vi "温度校准.vi"(7 "校准参数":u16(ring) caption="校准参数：" items=["pH", "DO", "浊度", "电导率", "叶绿素a", "藻密度", "ORP", "DO2", "氯化物"], 8 "error in (no error)":errorcluster caption="错误输入（无错误）", 11 "校准温度":sgl) -> (0 "error out":errorcluster caption="错误输出")   [LabVIEW 2016, in "斯坦道多参数.lvlib"]
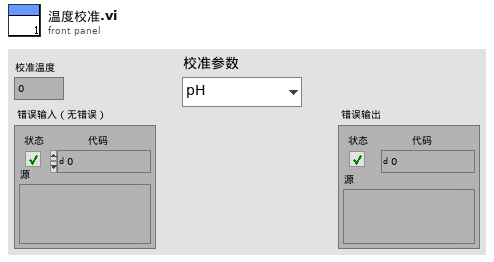
[diagram p1: front panel]
types:
  T1 = typedef "斯坦道多参数.lvlib/探头类型.ctl" = enum16{"禹山", "国弘", "纳清", "STD"}
  T2 = enum16{"null", "pH", "DO", "浊度", "电导率", "叶绿素a", "DO2", "藻密度"}
  T3 = enum16{"null", "pH", "DO", "浊度", "电导率", "叶绿素a", "DO2", "藻密度", "悬浮物"}
  T4 = enum16{"NULL", "pH", "Cond", "DO", "Turb", "ORP"}
  T5 = enum16{"NULL", "pH", "Cond", "DO", "Turb", "ORP", "6", "7", "8", "9", "氯化物"}
  T6 = enum16{"null", "pH", "DO", "浊度", "电导率", "叶绿素a", "藻密度"}
  T7 = enum16{"null", "pH", "DO", "浊度", "电导率", "叶绿素a", "藻密度", "氨氮"}
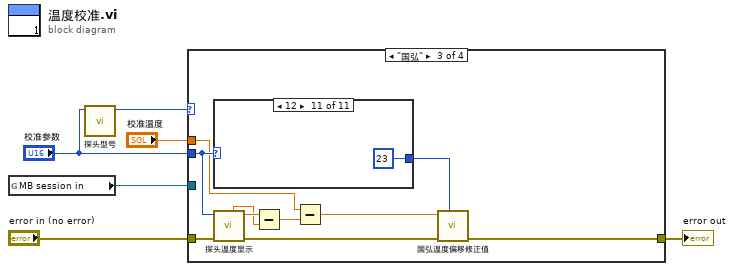
[diagram p0: block diagram]
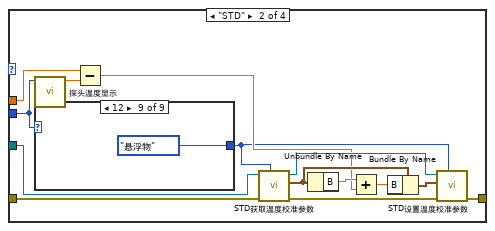
[diagram p3: hidden frame]
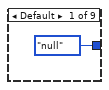
[diagram p4: hidden frame]
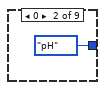
[diagram p5: hidden frame]
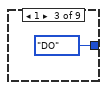
[diagram p6: hidden frame]
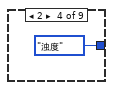
[diagram p7: hidden frame]
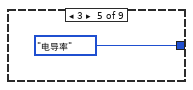
[diagram p8: hidden frame]
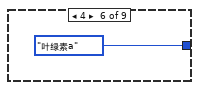
[diagram p9: hidden frame]
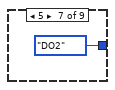
[diagram p10: hidden frame]
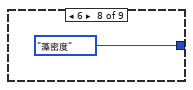
[diagram p11: hidden frame]
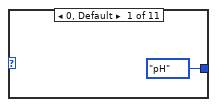
[diagram p12: hidden frame]
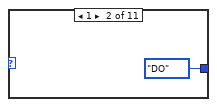
[diagram p13: hidden frame]
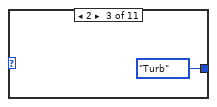
[diagram p14: hidden frame]
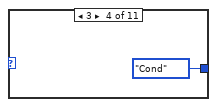
[diagram p15: hidden frame]
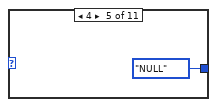
[diagram p16: hidden frame]
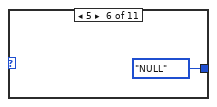
[diagram p17: hidden frame]
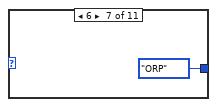
[diagram p18: hidden frame]
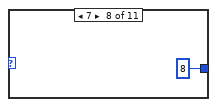
[diagram p19: hidden frame]
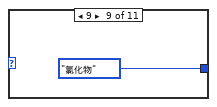
[diagram p20: hidden frame]
diagram:
  n1 = global read "多参数全局变量.vi" "MB session in"() -> (w4:refnum<class "MB_Master.lvclass">)
  n2 = call "探头型号.vi"("校准参数"="校准参数") -> ("探头型号"=w6:T1)  [unwired: 8 in, 2 out]
  n3 = case shown="\"国弘\"" w6 {
    tunnel: "校准参数" -> [_ w10 w36 w52]
    tunnel: w4 -> [_ w21 _ w54]
    tunnel: "error in (no error)" -> [w7 w8 w39 w56]
    tunnel: [w7 w11 w38 w55] -> w2
    tunnel: "校准温度" -> [_ w18 w32 w53]
    frame "禹山", Default {
    }
    frame "STD" {
      n4 = call "探头温度显示.vi"("校准参数"=w10) -> ("温度数据"=w19:sgl)  [unwired: 9 in, 1 out]
      n5 = case shown="12" w10 {
        tunnel: [T2."null" ("探头") T2."pH" ("探头") T2."DO" ("探头") T2."浊度" ("探头") T2."电导率" ("探头") T2."叶绿素a" ("探头") T2."DO2" ("探头") T2."藻密度" ("探头") T3."悬浮物" ("探头")] -> w9
        frame Default {
        }
        frame 0 {
        }
        frame 1 {
        }
        frame 2 {
        }
        frame 3 {
        }
        frame 4 {
        }
        frame 5 {
        }
        frame 6 {
        }
        frame 12 {
        }
      }
      n6 = Subtract(x=w18, y=w19) -> (x-y=w14:sgl)
      n7 = call "STD获取温度校准参数.vi"("探头"=w9, "error in (no error)"=w8, "MB session in"=w21) -> ("error out"=w17:errorcluster, "输出值"=w16:cluster{"K":sgl, "B":sgl}, "MB session out"=w20:refnum<class "MB_Master.lvclass">)  [unwired: 6 in]
      n8 = Unbundle By Name(w16) -> ("B"=w15:sgl)
      n9 = Add(x=w15, y=w14) -> (x+y=w13:sgl)
      n10 = Bundle By Name(cluster=w16, "B"=w13) -> (w12:cluster{"K":sgl, "B":sgl})
      n11 = call "STD设置温度校准参数.vi"("探头"=w9, "error in (no error)"=w17, "用户校准参数"=w12, "MB session in"=w20) -> ("error out"=w11:errorcluster)  [unwired: 6 in, 1 out]
    }
    frame "国弘" {
      n12 = case shown="12" w36 {
        tunnel: [T4."pH" ("探头") T4."DO" ("探头") T4."Turb" ("探头") T4."Cond" ("探头") T4."NULL" ("探头") T4."NULL" ("探头") T4."ORP" ("探头") 8 T5."氯化物" ("探头") 17 23] -> w37
        frame 0, Default {
        }
        frame 1 {
        }
        frame 2 {
        }
        frame 3 {
        }
        frame 4 {
        }
        frame 5 {
        }
        frame 6 {
        }
        frame 7 {
        }
        frame 9 {
        }
        frame 11 {
        }
        frame 12 {
        }
      }
      n13 = call "探头温度显示.vi"("校准参数"=w36) -> ("温度数据"=w35:sgl, "温度偏移修正值"=w34:sgl)  [unwired: 9 in]
      n14 = Subtract(x=w35, y=w34) -> (x-y=w33:sgl)
      n15 = Subtract(x=w32, y=w33) -> (x-y=w31:sgl)
      n16 = call "国弘温度偏移修正值.vi"("探头"=w37, "error in (no error)"=w39, "温度偏移修正值"=w31) -> ("error out"=w38:errorcluster)  [unwired: 7 in, 1 out]
    }
    frame "纳清" {
      n17 = case shown="7" w52 {
        tunnel: [T6."null" ("探头") T6."pH" ("探头") T6."DO" ("探头") T6."浊度" ("探头") T6."电导率" ("探头") T6."叶绿素a" ("探头") T6."藻密度" ("探头") T6."null" ("探头") T6."null" ("探头") T7."氨氮" ("探头") 17] -> w51
        frame Default {
        }
        frame 0 {
        }
        frame 1 {
        }
        frame 2 {
        }
        frame 3 {
        }
        frame 4 {
        }
        frame 5 {
        }
        frame 6 {
        }
        frame 7 {
        }
        frame 10 {
        }
        frame 11 {
        }
      }
      n18 = call "纳清_温度校准.vi"("探头"=w51, "error in (no error)"=w56, "校准温度"=w53, "MB session in"=w54) -> ("error out"=w55:errorcluster)  [unwired: 6 in, 1 out]
    }
  }
  "error out" <- w2
